vi "FTW-JSON-Core-GetFlattenedValue.vi"(0 "JSON Element":i64 format="%016x", 5 "Element Data Name":string, 7 "LabVIEW Type":T1, 9 "Element Default Value":variant, 11 "error in":errorcluster) -> (4 "Flattened Value":string, 15 "error out":errorcluster)   [LabVIEW 2013]
uses:
  Reflection/FTW-Reflection-Types.ctl
  FTW-JSON-Type.ctl
panel:
  # "Inputs"
  # "Outputs"
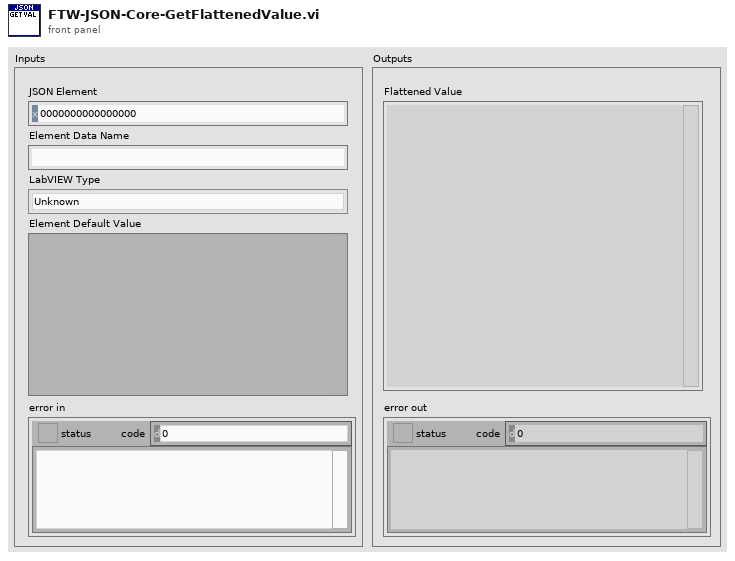
[diagram p1: front panel]
types:
  T1 = typedef "FTW-Reflection-Types.ctl" = enum16{"Unknown", "Void", "Array", "Cluster", "LVObject", "Boolean", "I8", "I16", "I32", "I64", "U8", "U16", "U32", "U64", "SGL", "DBL", "EXT", "CSG", "CDB", "CXT", "FXP", "EnumU8", "EnumU16", "EnumU32", "EnumU64", "SGLwithUnit", "DBLwithUnit", "EXTwithUnit", "CSGwithUnit", "CDBwithUnit", "CXTwithUnit", "String", "Path", "Picture", "Tag", "LVVariant", "Timestamp", "WaveformI8", "WaveformI16", "WaveformI32", "WaveformI64", "WaveformU8", "WaveformU16", "WaveformU32", "WaveformU64", "WaveformSGL", "WaveformDBL", "WaveformEXT", "WaveformCSG", "WaveformCDB", "WaveformCXT", "WaveformDigital", "WaveformUnknownType", "DigitalData", "DynamicData", "ExternalData", "FileByteStream", "TDMStream", "dotNET", "ActiveX", "VIServerReference", "VIReference", "ApplicationInstance", "Menu", "ConnectionDataSocket", "ConnectionVISA", "ConnectionBluetooth", "ConnectionIrDA", "ConnectionTCP", "ConnectionUDP", "ConnectionHTTPClient", "ConnectionFTP", "Occurrence", "Notifier", "Queue", "Rendezvous", "Semaphore", "RTFIFO", "EventPublisher", "EventRegistration", "EventCallback", "DataValueReference", "GenericClass", "GenericClassTag", "GenericClassDeepCopy", "GenericClassFlattened", "GenericClassTagFlattened", "GenericReferenceType", "WindowsRegistry", "OverloadedDatalogRef", "ReferenceUnknownType"}
  T2 = typedef "FTW-JSON-Type.ctl" = enum16{"Object", "Array", "String", "Integer", "Floating Point", "true", "false", "null", "undefined"}
  T3 = cluster{"Element Name":string, "Element Type":T1, "Element Value":variant}[]
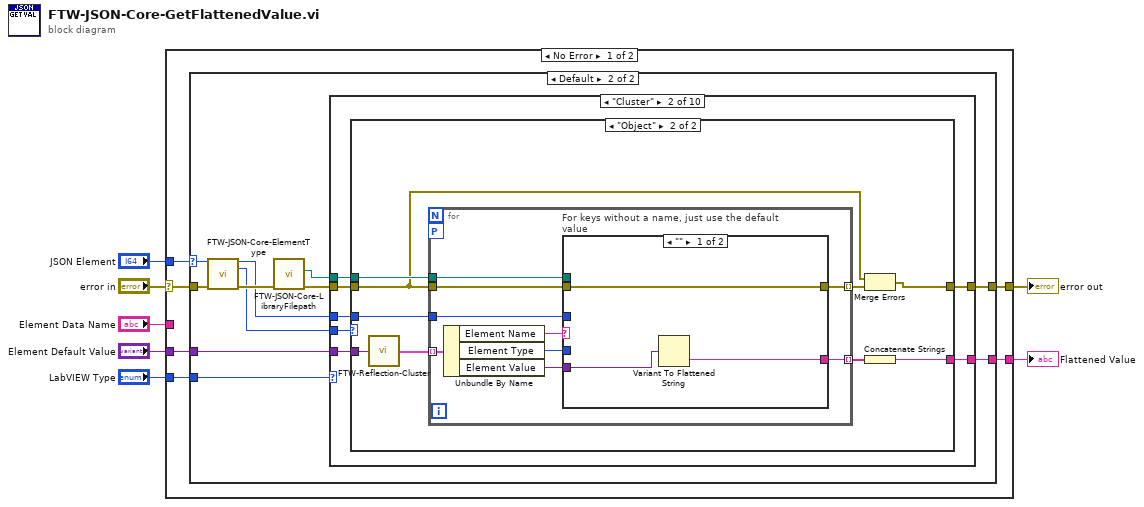
[diagram p0: block diagram]
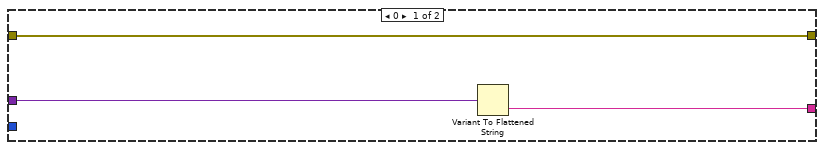
[diagram p2: hidden frame]
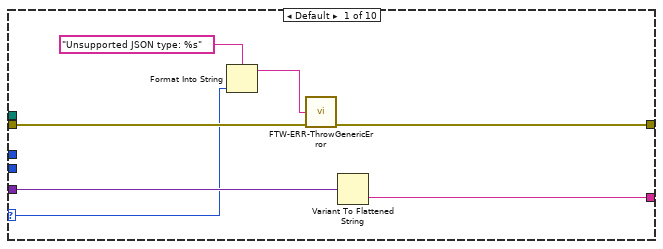
[diagram p3: hidden frame]
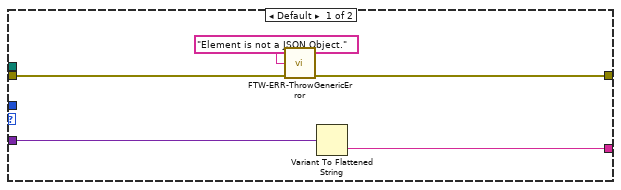
[diagram p4: hidden frame]
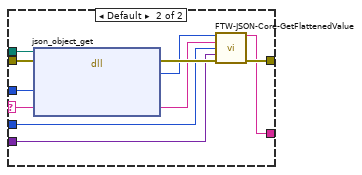
[diagram p5: hidden frame]
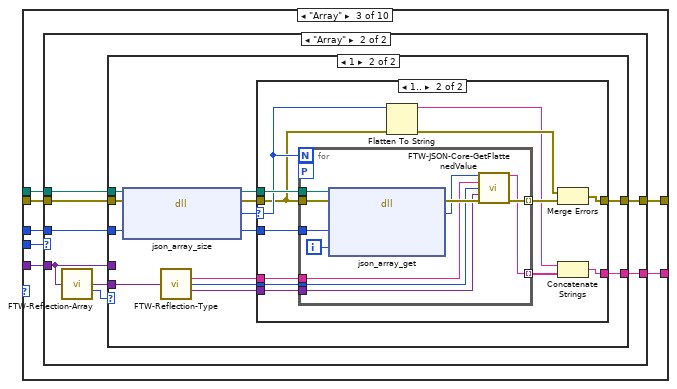
[diagram p6: hidden frame]
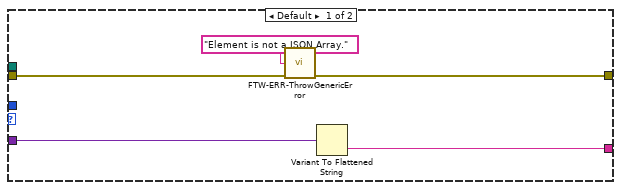
[diagram p7: hidden frame]
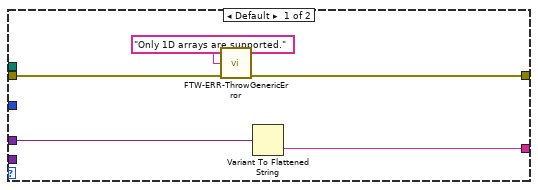
[diagram p8: hidden frame]
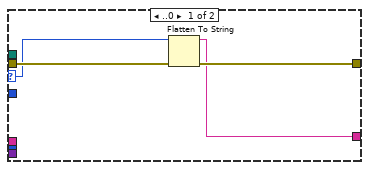
[diagram p9: hidden frame]
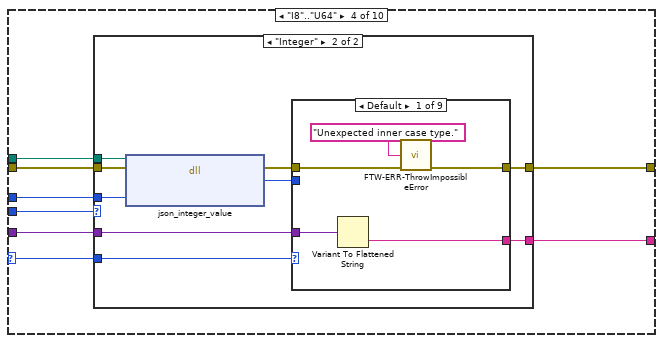
[diagram p10: hidden frame]
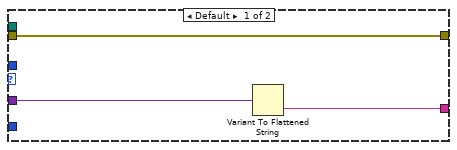
[diagram p11: hidden frame]
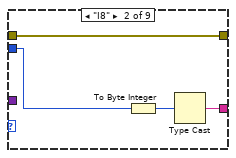
[diagram p12: hidden frame]
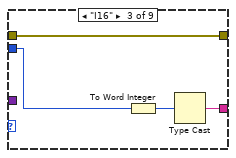
[diagram p13: hidden frame]
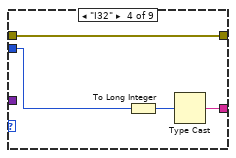
[diagram p14: hidden frame]
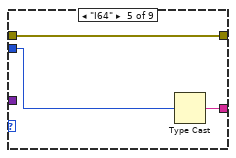
[diagram p15: hidden frame]
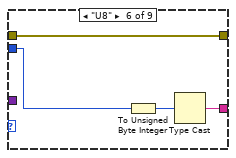
[diagram p16: hidden frame]
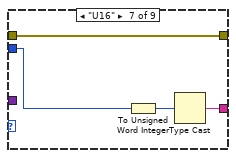
[diagram p17: hidden frame]
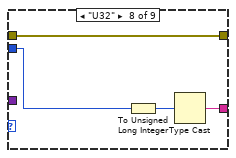
[diagram p18: hidden frame]
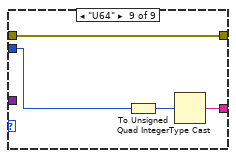
[diagram p19: hidden frame]
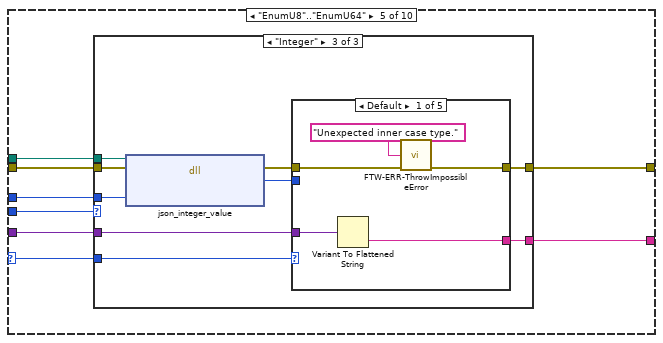
[diagram p20: hidden frame]
diagram:
  n1 = case shown="No Error" "error in" {
    selector: "error in" -> [w9 w439]
    tunnel: [w13 w439] -> w7
    tunnel: "JSON Element" -> [w8 _]
    tunnel: [w12 w437] -> w5
    tunnel: "LabVIEW Type" -> [w11 _]
    tunnel: "Element Default Value" -> [w10 w438]
    tunnel: "Element Data Name" -> [_ _]
    frame No Error {
      n2 = case shown="Default" w8 {
        selector: w8 -> [_ w17]
        tunnel: [w14 w27] -> w13
        tunnel: [w15 w26] -> w12
        tunnel: w11 -> [_ w23]
        tunnel: w10 -> [w16 w22]
        tunnel: w9 -> [w14 w21]
        frame 0 {
          n3 = Variant To Flattened String(Variant=w16) -> (data string=w15:string)  [unwired: 1 out]
        }
        frame Default {
          n4 = call "FTW-JSON-Core-ElementType.vi"("JSON Element"=w17, "error in"=w21) -> ("JSON Element out"=w19:i64, "JSON Type"=w18:T2, "error out"=w20:errorcluster)  [unwired: 11 in]
          n5 = call "FTW-JSON-Core-LibraryFilepath.vi"("error in"=w20) -> ("error out"=w25:errorcluster, "JSON Library Filepath"=w24:path)  [unwired: 9 in]
          n6 = case shown="\"Cluster\"" w23 {
            selector: w23 -> [w28 _ _ w148 w204 w287 _ w350 _ _]
            tunnel: [w31 w37 w83 w145 w201 w284 w320 w347 w393 w424] -> w27
            tunnel: [w29 w40 w84 w150 w206 w289 w324 w352 w397 w427] -> w26
            tunnel: w25 -> [w32 w36 w82 w151 w207 w290 w325 w353 w398 w428]
            tunnel: w24 -> [_ w39 w80 w152 w208 w291 w326 w354 w399 _]
            tunnel: w19 -> [_ w38 w79 w147 w203 w286 w322 w349 w395 _]
            tunnel: w22 -> [w30 w41 w85 w149 w205 w288 w323 w351 w396 w426]
            tunnel: w18 -> [_ w35 w81 w146 w202 w285 w321 w348 w394 w425]
            frame Default {
              n7 = Format Into String(format string="Unsupported JSON type: %s", w28) -> (resulting string=w34:string)  [unwired: 2 in, 1 out]
              n8 = call "FTW-ERR-ThrowGenericError.vi"("Error Message"=w34, "error in"=w32) -> ("error out"=w31:errorcluster)  [unwired: 13 in]
              n9 = Variant To Flattened String(Variant=w30) -> (data string=w29:string)  [unwired: 1 out]
            }
            frame "Cluster" {
              n10 = case shown="\"Object\"" w35 {
                tunnel: w41 -> [w44 w54]
                tunnel: [w43 w52] -> w40
                tunnel: w39 -> [_ w51]
                tunnel: w38 -> [_ w49]
                tunnel: [w45 w48] -> w37
                tunnel: w36 -> [w46 w47]
                frame Default {
                  n11 = call "FTW-ERR-ThrowGenericError.vi"("Error Message"="Element is not a JSON Object.", "error in"=w46) -> ("error out"=w45:errorcluster)  [unwired: 13 in]
                  n12 = Variant To Flattened String(Variant=w44) -> (data string=w43:string)  [unwired: 1 out]
                }
                frame "Object" {
                  n13 = call "FTW-Reflection-Cluster.vi"("Cluster"=w54) -> ("Cluster Elements"=w55:T3)  [unwired: 14 in]
                  n14 = for {
                    tunnel: w55 -> [w63] mode=indexing
                    tunnel: [w60] -> w53 mode=indexing
                    tunnel: w51 -> [w57]
                    tunnel: w49 -> [w56]
                    tunnel: w47 -> [w64]
                    tunnel: [w58] -> w50 mode=indexing
                    workers-P: _ -> [_]
                    n15 = Unbundle By Name(w63) -> ("Element Name"=w62:string, "Element Type"=w59:T1, "Element Value"=w61:variant)
                    n16 = case "For keys without a name, just use the default value" shown="\"\"" w62 {
                      selector: w62 -> [_ w74]
                      tunnel: w57 -> [_ w77]
                      tunnel: w64 -> [w65 w76]
                      tunnel: w61 -> [w67 w70]
                      tunnel: [w66 w71] -> w60
                      tunnel: w56 -> [_ w75]
                      tunnel: w59 -> [_ w69]
                      tunnel: [w65 w72] -> w58
                      frame "" {
                        n17 = Variant To Flattened String(Variant=w67) -> (data string=w66:string)  [unwired: 1 out]
                      }
                      frame Default {
                        n18 = dll-call lib="?" fn="json_object_get"(path in=w77, error in=w76, "JSON Object Pointer"=w75, "Element Key"=w74) -> (error out=w78:errorcluster, "JSON Element Pointer"=w73:i64, "Element Key"=w68:string)  [unwired: 2 in, 1 out]
                        n19 = call "FTW-JSON-Core-GetFlattenedValue.vi"("JSON Element"=w73, "Element Data Name"=w68, "LabVIEW Type"=w69, "Element Default Value"=w70, "error in"=w78) -> ("Flattened Value"=w71:string, "error out"=w72:errorcluster)  [unwired: 9 in]
                      }
                    }
                  }
                  n20 = Merge Errors(w47, w50) -> (w48:errorcluster)
                  n21 = Concatenate Strings(w53) -> (w52:string)
                }
              }
            }
            frame "Array" {
              n22 = case shown="\"Array\"" w81 {
                tunnel: w85 -> [w88 w91]
                tunnel: [w87 w98] -> w84
                tunnel: [w86 w97] -> w83
                tunnel: w82 -> [w89 w96]
                tunnel: w80 -> [_ w93]
                tunnel: w79 -> [_ w92]
                frame Default {
                  n23 = call "FTW-ERR-ThrowGenericError.vi"("Error Message"="Element is not a JSON Array.", "error in"=w89) -> ("error out"=w86:errorcluster)  [unwired: 13 in]
                  n24 = Variant To Flattened String(Variant=w88) -> (data string=w87:string)  [unwired: 1 out]
                }
                frame "Array" {
                  n25 = call "FTW-Reflection-Array.vi"("Array"=w91) -> ("Default Array Element"=w95:variant, "Number of Dimensions"=w94:i32)  [unwired: 13 in]
                  n26 = case shown="1" w94 {
                    tunnel: [w100 w116] -> w98
                    tunnel: [w101 w115] -> w97
                    tunnel: w96 -> [w102 w114]
                    tunnel: w95 -> [_ w108]
                    tunnel: w93 -> [_ w113]
                    tunnel: w92 -> [_ w112]
                    tunnel: w91 -> [w99 _]
                    frame Default {
                      n27 = call "FTW-ERR-ThrowGenericError.vi"("Error Message"="Only 1D arrays are supported.", "error in"=w102) -> ("error out"=w101:errorcluster)  [unwired: 13 in]
                      n28 = Variant To Flattened String(Variant=w99) -> (data string=w100:string)  [unwired: 1 out]
                    }
                    frame 1 {
                      n29 = dll-call lib="?" fn="json_array_size"(path in=w113, error in=w114, "Array Pointer"=w112) -> (path out=w111:path, error out=w109:errorcluster, "Array Size"=w105:i32, "Array Pointer"=w110:i64)  [unwired: 1 in]
                      n30 = call "FTW-Reflection-Type.vi"("Anything"=w108) -> ("Data Name"=w104:string, "LabVIEW Type"=w107:T1, "Variant Type and Value"=w106:variant)  [unwired: 12 in]
                      n31 = case shown="1.." w105 {
                        selector: w105 -> [w117 w125]
                        tunnel: [w119 w133] -> w116
                        tunnel: [w120 w132] -> w115
                        tunnel: w111 -> [_ w131]
                        tunnel: w110 -> [_ w130]
                        tunnel: w109 -> [w118 w122]
                        tunnel: w107 -> [_ w128]
                        tunnel: w106 -> [_ w127]
                        tunnel: w104 -> [_ w121]
                        frame ..0 {
                          n32 = Flatten To String(anything=w117, error in (no error)=w118) -> (data string=w119:string, error out=w120:errorcluster)  [unwired: 2 in, 1 out]
                        }
                        frame 1.. {
                          n33 = for {
                            N: w125 -> [_]
                            tunnel: w131 -> [w143]
                            tunnel: w130 -> [w141]
                            workers-P: _ -> [_]
                            tunnel: w122 -> [w142]
                            tunnel: [w139] -> w129 mode=indexing
                            tunnel: w128 -> [w135]
                            tunnel: w127 -> [w136]
                            tunnel: [w137] -> w126 mode=indexing
                            tunnel: w121 -> [w134]
                            i -> [w140]
                            n34 = dll-call lib="?" fn="json_array_get"(path in=w143, error in=w142, "Array Pointer"=w141, "Index"=w140) -> (error out=w144:errorcluster, "Array Element"=w138:i64)  [unwired: 3 in, 1 out]
                            n35 = call "FTW-JSON-Core-GetFlattenedValue.vi"("JSON Element"=w138, "Element Data Name"=w134, "LabVIEW Type"=w135, "Element Default Value"=w136, "error in"=w144) -> ("Flattened Value"=w137:string, "error out"=w139:errorcluster)  [unwired: 9 in]
                          }
                          n36 = Flatten To String(anything=w125, error in (no error)=w122) -> (data string=w123:string, error out=w124:errorcluster)  [unwired: 2 in, 1 out]
                          n37 = Merge Errors(w124, w129) -> (w132:errorcluster)
                          n38 = Concatenate Strings(w123, w126) -> (w133:string)
                        }
                      }
                    }
                  }
                }
              }
            }
            frame "I8".."U64" {
              n39 = case shown="\"Integer\"" w146 {
                tunnel: w152 -> [_ w164]
                tunnel: w147 -> [_ w163]
                tunnel: w151 -> [w153 w162]
                tunnel: w149 -> [w155 w156]
                tunnel: [w154 w157] -> w150
                tunnel: [w153 w160] -> w145
                tunnel: w148 -> [_ w161]
                frame Default {
                  n40 = Variant To Flattened String(Variant=w155) -> (data string=w154:string)  [unwired: 1 out]
                }
                frame "Integer" {
                  n41 = dll-call lib="?" fn="json_integer_value"(path in=w164, error in=w162, "JSON Element Pointer"=w163) -> (error out=w159:errorcluster, "I64 Value"=w158:i64)  [unwired: 2 in, 1 out]
                  n42 = case shown="Default" w161 {
                    tunnel: [w168 w173 w177 w181 w184 w188 w192 w196 w200] -> w160
                    tunnel: w159 -> [w169 w173 w177 w181 w184 w188 w192 w196 w200]
                    tunnel: w158 -> [_ w171 w175 w179 w182 w186 w190 w194 w198]
                    tunnel: [w165 w172 w176 w180 w183 w187 w191 w195 w199] -> w157
                    tunnel: w156 -> [w166 _ _ _ _ _ _ _ _]
                    frame Default {
                      n43 = Variant To Flattened String(Variant=w166) -> (data string=w165:string)  [unwired: 1 out]
                      n44 = call "FTW-ERR-ThrowImpossibleError.vi"("Reason this error should never happen"="Unexpected inner case type.", "error in"=w169) -> ("error out"=w168:errorcluster)  [unwired: 13 in]
                    }
                    frame "I8" {
                      n45 = To Byte Integer(number=w171) -> (8bit integer=w170:i8)
                      n46 = Type Cast(x=w170) -> (*(type *) &x=w172:string)  [unwired: 1 in]
                    }
                    frame "I16" {
                      n47 = To Word Integer(number=w175) -> (16bit integer=w174:i16)
                      n48 = Type Cast(x=w174) -> (*(type *) &x=w176:string)  [unwired: 1 in]
                    }
                    frame "I32" {
                      n49 = To Long Integer(number=w179) -> (32bit integer=w178:i32)
                      n50 = Type Cast(x=w178) -> (*(type *) &x=w180:string)  [unwired: 1 in]
                    }
                    frame "I64" {
                      n51 = Type Cast(x=w182) -> (*(type *) &x=w183:string)  [unwired: 1 in]
                    }
                    frame "U8" {
                      n52 = To Unsigned Byte Integer(number=w186) -> (unsigned 8bit integer=w185:u8)
                      n53 = Type Cast(x=w185) -> (*(type *) &x=w187:string)  [unwired: 1 in]
                    }
                    frame "U16" {
                      n54 = To Unsigned Word Integer(number=w190) -> (unsigned 16bit integer=w189:u16)
                      n55 = Type Cast(x=w189) -> (*(type *) &x=w191:string)  [unwired: 1 in]
                    }
                    frame "U32" {
                      n56 = To Unsigned Long Integer(number=w194) -> (unsigned 32bit integer=w193:u32)
                      n57 = Type Cast(x=w193) -> (*(type *) &x=w195:string)  [unwired: 1 in]
                    }
                    frame "U64" {
                      n58 = To Unsigned Quad Integer(1:w198) -> (0:w197:u64)
                      n59 = Type Cast(x=w197) -> (*(type *) &x=w199:string)  [unwired: 1 in]
                    }
                  }
                }
              }
            }
            frame "EnumU8".."EnumU64" {
              n60 = case shown="\"Integer\"" w202 {
                tunnel: w208 -> [_ w220 w260]
                tunnel: w203 -> [_ w219 w258]
                tunnel: w207 -> [w209 w218 w259]
                tunnel: w205 -> [w211 w212 w257]
                tunnel: [w210 w213 w254] -> w206
                tunnel: [w209 w216 w255] -> w201
                tunnel: w204 -> [_ w217 w256]
                frame Default {
                  n61 = Variant To Flattened String(Variant=w211) -> (data string=w210:string)  [unwired: 1 out]
                }
                frame "String" {
                  n62 = dll-call lib="?" fn="json_string_value"(path in=w220, error in=w218, "JSON Element Pointer"=w219) -> (error out=w215:errorcluster, "String Value"=w214:string)  [unwired: 2 in, 1 out]
                  n63 = case shown="Default" w217 {
                    tunnel: [w224 w232 w239 w246 w253] -> w216
                    tunnel: w215 -> [w225 w232 w239 w246 w253]
                    tunnel: w214 -> [_ w229 w236 w243 w250]
                    tunnel: [w221 w228 w235 w242 w249] -> w213
                    tunnel: w212 -> [w222 w231 w238 w245 w252]
                    frame Default {
                      n64 = Variant To Flattened String(Variant=w222) -> (data string=w221:string)  [unwired: 1 out]
                      n65 = call "FTW-ERR-ThrowImpossibleError.vi"("Reason this error should never happen"="Unexpected inner case type.", "error in"=w225) -> ("error out"=w224:errorcluster)  [unwired: 13 in]
                    }
                    frame "EnumU8" {
                      n66 = call "FTW-Reflection-Enum.vi"("Enum"=w231) -> ("Enum Items"=w230:string[])  [unwired: 12 in, 2 out]
                      n67 = Search 1D Array(1D array=w230, element=w229) -> (index of element=w227:i32)  [unwired: 1 in]
                      n68 = To Unsigned Byte Integer(number=w227) -> (unsigned 8bit integer=w226:u8)
                      n69 = Type Cast(x=w226) -> (*(type *) &x=w228:string)  [unwired: 1 in]
                    }
                    frame "EnumU16" {
                      n70 = call "FTW-Reflection-Enum.vi"("Enum"=w238) -> ("Enum Items"=w237:string[])  [unwired: 12 in, 2 out]
                      n71 = Search 1D Array(1D array=w237, element=w236) -> (index of element=w234:i32)  [unwired: 1 in]
                      n72 = To Unsigned Word Integer(number=w234) -> (unsigned 16bit integer=w233:u16)
                      n73 = Type Cast(x=w233) -> (*(type *) &x=w235:string)  [unwired: 1 in]
                    }
                    frame "EnumU32" {
                      n74 = call "FTW-Reflection-Enum.vi"("Enum"=w245) -> ("Enum Items"=w244:string[])  [unwired: 12 in, 2 out]
                      n75 = Search 1D Array(1D array=w244, element=w243) -> (index of element=w241:i32)  [unwired: 1 in]
                      n76 = To Unsigned Long Integer(number=w241) -> (unsigned 32bit integer=w240:u32)
                      n77 = Type Cast(x=w240) -> (*(type *) &x=w242:string)  [unwired: 1 in]
                    }
                    frame "EnumU64" {
                      n78 = call "FTW-Reflection-Enum.vi"("Enum"=w252) -> ("Enum Items"=w251:string[])  [unwired: 12 in, 2 out]
                      n79 = Search 1D Array(1D array=w251, element=w250) -> (index of element=w248:i32)  [unwired: 1 in]
                      n80 = To Unsigned Quad Integer(1:w248) -> (0:w247:u64)
                      n81 = Type Cast(x=w247) -> (*(type *) &x=w249:string)  [unwired: 1 in]
                    }
                  }
                }
                frame "Integer" {
                  n82 = dll-call lib="?" fn="json_integer_value"(path in=w260, error in=w259, "JSON Element Pointer"=w258) -> (error out=w262:errorcluster, "I64 Value"=w261:i64)  [unwired: 2 in, 1 out]
                  n83 = case shown="Default" w256 {
                    tunnel: [w266 w271 w275 w279 w283] -> w255
                    tunnel: w262 -> [w267 w271 w275 w279 w283]
                    tunnel: w261 -> [_ w269 w273 w277 w281]
                    tunnel: [w263 w270 w274 w278 w282] -> w254
                    tunnel: w257 -> [w264 _ _ _ _]
                    frame Default {
                      n84 = Variant To Flattened String(Variant=w264) -> (data string=w263:string)  [unwired: 1 out]
                      n85 = call "FTW-ERR-ThrowImpossibleError.vi"("Reason this error should never happen"="Unexpected inner case type.", "error in"=w267) -> ("error out"=w266:errorcluster)  [unwired: 13 in]
                    }
                    frame "EnumU8" {
                      n86 = To Unsigned Byte Integer(number=w269) -> (unsigned 8bit integer=w268:u8)
                      n87 = Type Cast(x=w268) -> (*(type *) &x=w270:string)  [unwired: 1 in]
                    }
                    frame "EnumU16" {
                      n88 = To Unsigned Word Integer(number=w273) -> (unsigned 16bit integer=w272:u16)
                      n89 = Type Cast(x=w272) -> (*(type *) &x=w274:string)  [unwired: 1 in]
                    }
                    frame "EnumU32" {
                      n90 = To Unsigned Long Integer(number=w277) -> (unsigned 32bit integer=w276:u32)
                      n91 = Type Cast(x=w276) -> (*(type *) &x=w278:string)  [unwired: 1 in]
                    }
                    frame "EnumU64" {
                      n92 = To Unsigned Quad Integer(1:w281) -> (0:w280:u64)
                      n93 = Type Cast(x=w280) -> (*(type *) &x=w282:string)  [unwired: 1 in]
                    }
                  }
                }
              }
            }
            frame "SGL".."EXT" {
              n94 = case shown="\"Integer\", \"Floating Point\"" w285 {
                tunnel: w291 -> [_ w303]
                tunnel: w286 -> [_ w302]
                tunnel: w290 -> [w292 w301]
                tunnel: w288 -> [w294 w295]
                tunnel: [w293 w296] -> w289
                tunnel: [w292 w299] -> w284
                tunnel: w287 -> [_ w300]
                frame Default {
                  n95 = Variant To Flattened String(Variant=w294) -> (data string=w293:string)  [unwired: 1 out]
                }
                frame "Integer", "Floating Point" {
                  n96 = dll-call lib="?" fn="json_number_value"(path in=w303, error in=w301, "JSON Element Pointer"=w302) -> (error out=w298:errorcluster, "DBL Value"=w297:dbl)  [unwired: 2 in, 1 out]
                  n97 = case shown="Default" w300 {
                    tunnel: [w307 w312 w315 w319] -> w299
                    tunnel: w298 -> [w308 w312 w315 w319]
                    tunnel: w297 -> [_ w309 w313 w317]
                    tunnel: [w304 w311 w314 w318] -> w296
                    tunnel: w295 -> [w305 _ _ _]
                    frame Default {
                      n98 = Variant To Flattened String(Variant=w305) -> (data string=w304:string)  [unwired: 1 out]
                      n99 = call "FTW-ERR-ThrowImpossibleError.vi"("Reason this error should never happen"="Unexpected inner case type.", "error in"=w308) -> ("error out"=w307:errorcluster)  [unwired: 13 in]
                    }
                    frame "SGL" {
                      n100 = To Single Precision Float(number=w309) -> (single precision float=w310:sgl)
                      n101 = Type Cast(x=w310) -> (*(type *) &x=w311:string)  [unwired: 1 in]
                    }
                    frame "DBL" {
                      n102 = Type Cast(x=w313) -> (*(type *) &x=w314:string)  [unwired: 1 in]
                    }
                    frame "EXT" {
                      n103 = To Extended Precision Float(1:w317) -> (0:w316:ext)
                      n104 = Type Cast(x=w316) -> (*(type *) &x=w318:string)  [unwired: 1 in]
                    }
                  }
                }
              }
            }
            frame "Timestamp" {
              n105 = case shown="\"String\"" w321 {
                tunnel: w326 -> [_ w336 w340]
                tunnel: w322 -> [_ w335 w339]
                tunnel: w325 -> [w327 w334 w341]
                tunnel: w323 -> [w329 _ _]
                tunnel: [w328 w332 w346] -> w324
                tunnel: [w327 w333 w343] -> w320
                frame Default {
                  n106 = Variant To Flattened String(Variant=w329) -> (data string=w328:string)  [unwired: 1 out]
                }
                frame "Floating Point" {
                  n107 = dll-call lib="?" fn="json_number_value"(path in=w336, error in=w334, "JSON Element Pointer"=w335) -> (error out=w333:errorcluster, "DBL Value"=w331:dbl)  [unwired: 2 in, 1 out]
                  n108 = To Time Stamp(1:w331) -> (0:w330:timestamp)
                  n109 = Type Cast(x=w330) -> (*(type *) &x=w332:string)  [unwired: 1 in]
                }
                frame "String" {
                  n110 = dll-call lib="?" fn="json_string_value"(path in=w340, error in=w341, "JSON Element Pointer"=w339) -> (error out=w343:errorcluster, "String Value"=w342:string)  [unwired: 2 in, 1 out]
                  n111 = Scan From String(format string="%^<%Y-%m-%dT%H:%M:%S%3uZ>T", input string=w342, default 1=timestamp(0 s since 1904-01-01) ("LabVIEW Timestamp")) -> (error out=w345:errorcluster, output 1=w344:timestamp)  [unwired: 2 in, 2 out]
                  n112 = call "FTW-ERR-Clear.vi"("error to snuff"=w345) -> ()  [unwired: 1 out]
                  n113 = Type Cast(x=w344) -> (*(type *) &x=w346:string)  [unwired: 1 in]
                }
              }
            }
            frame "String".."Tag", "ConnectionVISA" {
              n114 = case shown="\"String\"" w348 {
                tunnel: w354 -> [_ w366]
                tunnel: w349 -> [_ w365]
                tunnel: w353 -> [w355 w364]
                tunnel: w351 -> [w357 w358]
                tunnel: [w356 w359] -> w352
                tunnel: [w355 w362] -> w347
                tunnel: w350 -> [_ w363]
                frame Default {
                  n115 = Variant To Flattened String(Variant=w357) -> (data string=w356:string)  [unwired: 1 out]
                }
                frame "String" {
                  n116 = dll-call lib="?" fn="json_string_value"(path in=w366, error in=w364, "JSON Element Pointer"=w365) -> (error out=w361:errorcluster, "String Value"=w360:string)  [unwired: 2 in, 1 out]
                  n117 = case shown="\"Tag\"" w363 {
                    tunnel: [w370 w374 w378 w382 w387 w392] -> w362
                    tunnel: w361 -> [w371 w375 w379 w383 w388 w392]
                    tunnel: w360 -> [_ w373 w377 w381 w386 w391]
                    tunnel: [w367 w372 w376 w380 w385 w390] -> w359
                    tunnel: w358 -> [w368 _ _ _ _ _]
                    frame Default {
                      n118 = Variant To Flattened String(Variant=w368) -> (data string=w367:string)  [unwired: 1 out]
                      n119 = call "FTW-ERR-ThrowImpossibleError.vi"("Reason this error should never happen"="Unexpected inner case type.", "error in"=w371) -> ("error out"=w370:errorcluster)  [unwired: 13 in]
                    }
                    frame "String" {
                      n120 = Flatten To String(anything=w373, error in (no error)=w375) -> (data string=w372:string, error out=w374:errorcluster)  [unwired: 2 in, 1 out]
                    }
                    frame "Tag" {
                      n121 = Flatten To String(anything=w377, error in (no error)=w379) -> (data string=w376:string, error out=w378:errorcluster)  [unwired: 2 in, 1 out]
                    }
                    frame "ConnectionVISA" {
                      n122 = Flatten To String(anything=w381, error in (no error)=w383) -> (data string=w380:string, error out=w382:errorcluster)  [unwired: 2 in, 1 out]
                    }
                    frame "Path" {
                      n123 = String To Path(string=w386) -> (path=w384:path)
                      n124 = Flatten To String(anything=w384, error in (no error)=w388) -> (data string=w385:string, error out=w387:errorcluster)  [unwired: 2 in, 1 out]
                    }
                    frame "Picture" {
                      n125 = call "FTW-STR-Encode-Base64.vi"("Input"=w391, "Direction"=enum16{"Encode", "Decode"}."Decode") -> ("Output"=w390:string)
                    }
                  }
                }
              }
            }
            frame "FileByteStream".."ConnectionDataSocket", "ConnectionBluetooth".."ReferenceUnknownType" {
              n126 = case shown="\"String\"" w394 {
                tunnel: w399 -> [_ w414]
                tunnel: w395 -> [_ w413]
                tunnel: w398 -> [w400 w412]
                tunnel: w396 -> [w402 w407]
                tunnel: [w401 w409] -> w397
                tunnel: [w400 w405] -> w393
                frame Default {
                  n127 = Variant To Flattened String(Variant=w402) -> (data string=w401:string)  [unwired: 1 out]
                }
                frame "String" {
                  w410 = "0x%16x"  # Reference Format
                  n128 = dll-call lib="?" fn="json_string_value"(path in=w414, error in=w412, "JSON Element Pointer"=w413) -> (error out=w404:errorcluster, "String Value"=w411:string, "JSON Element Pointer"=w403:i64)  [unwired: 1 in, 1 out]
                  n129 = Scan From String(format string=w410, input string=w411, error in=w404, default 1=w403) -> (error out=w406:errorcluster, output 1=w408:i64)  [unwired: 1 in, 2 out]
                  n130 = case shown="No Error" w406 {
                    selector: w406 -> [w415 _]
                    tunnel: [w419 w422] -> w409
                    tunnel: w408 -> [w418 _]
                    tunnel: w407 -> [_ w423]
                    tunnel: [w415 w421] -> w405
                    frame No Error {
                      n131 = Type Cast(type=refnum<k0> refnum, x=w418) -> (*(type *) &x=w417:refnum<k0>)
                      n132 = Type Cast(x=w417) -> (*(type *) &x=w419:string)  [unwired: 1 in]
                    }
                    frame Error {
                      n133 = Variant To Flattened String(Variant=w423) -> (data string=w422:string)  [unwired: 1 out]
                      n134 = call "FTW-ERR-ThrowGenericError.vi"("Error Message"="Unexpected reference format.") -> ("error out"=w421:errorcluster)  [unwired: 14 in]
                    }
                  }
                }
              }
            }
            frame "Boolean" {
              n135 = case shown="\"true\", \"false\"" w425 {
                selector: w425 -> [_ w434]
                tunnel: w428 -> [w429 w435]
                tunnel: w426 -> [w431 _]
                tunnel: [w430 w436] -> w427
                tunnel: [w429 w435] -> w424
                frame Default {
                  n136 = Variant To Flattened String(Variant=w431) -> (data string=w430:string)  [unwired: 1 out]
                }
                frame "true", "false" {
                  n137 = Equal?(x=w434, y=FTW-JSON-Type."true" ("x")) -> (x = y?=w432:bool)
                  n138 = Type Cast(x=w432) -> (*(type *) &x=w436:string)  [unwired: 1 in]
                }
              }
            }
          }
        }
      }
    }
    frame Error {
      n139 = Variant To Flattened String(Variant=w438) -> (data string=w437:string)  [unwired: 1 out]
    }
  }
  "error out" <- w7
  "Flattened Value" <- w5
